vi "LVClass_CameraSet WriteFile CameraParametersSetup.vi"(0 "CameraSet in":refnum<class "CameraSet.lvclass">, 11 "error in (no error)":errorcluster) -> (4 "CameraSet out":refnum<class "CameraSet.lvclass">, 15 "error out":errorcluster)   [LabVIEW 2020, in "CameraSet.lvclass"]
uses:
  CameraSet.lvclass
  CameraSet.lvclass/CameraSet.ctl
  Write to XML File(string).vi
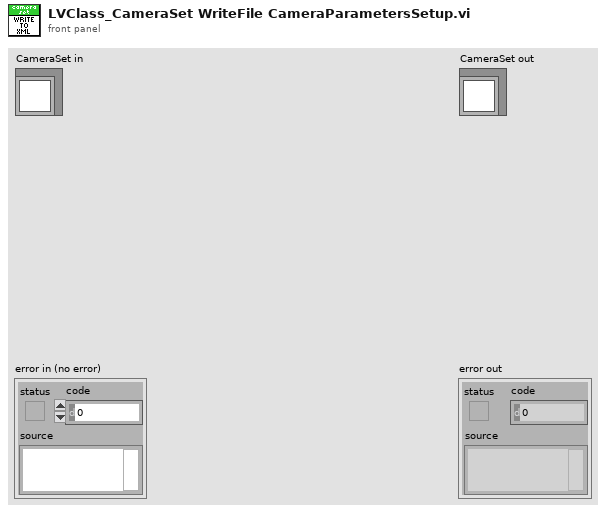
[diagram p1: front panel]
types:
  T1 = typedef "CameraParametersSetup.ctl" = cluster{"Name":string, "Type":T2, "Value":dbl, "BooleanValue":bool, "StringValue":string}
  T2 = typedef "CameraParameters_Type.ctl" = enum16{"Integer", "Real", "String", "Boolean"}
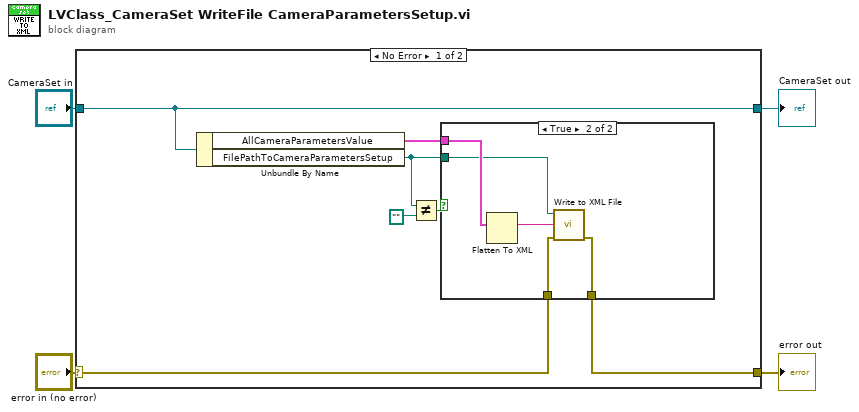
[diagram p0: block diagram]
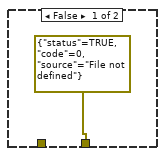
[diagram p2: hidden frame]
diagram:
  n1 = case shown="No Error" "error in (no error)" {
    selector: "error in (no error)" -> [w9 w19]
    tunnel: [w8 w19] -> w3
    tunnel: [w11 w18] -> w1
    tunnel: "CameraSet in" -> [w11 w18]
    frame No Error {
      n2 = Unbundle By Name(w11) -> ("AllCameraParametersValue"=w10:T1[], "FilePathToCameraParametersSetup"=w5:path)
      n3 = Not Equal?(x=w5, y=path "") -> (x != y?=w6:bool)
      n4 = case shown="True" w6 {
        tunnel: w10 -> [_ w17]
        tunnel: w5 -> [_ w15]
        tunnel: w9 -> [_ w14]
        tunnel: [errorcluster {"status"=TRUE, "code"=0, "source"="File not defined"} ("error out") w13] -> w8
        frame False {
        }
        frame True {
          n5 = Flatten To XML(6:w17) -> (2:w16:string)
          n6 = call-poly "Write to XML File.vi"("error in (no error)"=w14, "XML Input"=w16, "XML File Path"=w15) -> ("error out"=w13:errorcluster)  [unwired: 6 in, 2 out]
        }
      }
    }
    frame Error {
    }
  }
  "error out" <- w3
  "CameraSet out" <- w1
